vi "Module Type.vi"(11 "HTTP Command Bridge in":refnum<class "HTTP Command Bridge.lvclass">) -> (2 "Module Type":string)   [LabVIEW 2020, in "Volatus.lvlib" / "HTTP Command Bridge.lvclass"]
uses:
  HTTP Command Bridge.lvclass
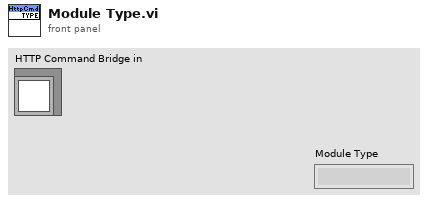
[diagram p1: front panel]
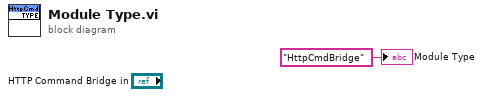
[diagram p0: block diagram]
diagram:
  "Module Type" <- "HttpCmdBridge" ("Module Type")
